vi "json Insert - String Path.vi"(8 "error in (no error)":errorcluster, 9 "anything":variant, 10 "path":string, 11 "JSON Document in":refnum<class "JSON Document.lvclass">) -> (0 "error out":errorcluster, 1 "replaced?":bool, 3 "JSON Document out":refnum<class "JSON Document.lvclass">)   [LabVIEW 2016, in "JSON Document.lvclass"]
uses:
  JSON Document.lvclass
  json query/json Query - string path.vi
  <vilib>/Utility/Data Type/NI_Data Type.lvlib
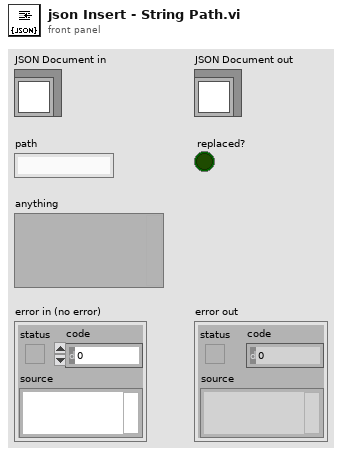
[diagram p1: front panel]
types:
  T1 = typedef "NI_Data Type.lvlib/Data Type.ctl" = enum8{"Invalid Type", "Void", "I8", "I16", "I32", "I64", "U8", "U16", "U32", "U64", "Single Float", "Double Float", "Extended Float", "Single Complex", "Double Complex", "Extended Complex", "Enum U8", "Enum U16", "Enum U32", "Enum U64", "Single Float With Unit", "Double Float With Unit", "Extended Float With Unit", "Single Complex with Unit", "Double Complex with Unit", "Extended Complex with Unit", "Boolean", "String", "Path", "Picture", "Tag", "Array", "Cluster", "Variant", "LV Variant", "Waveform", "Timestamp", "Digital Waveform", "Digital Data", "ExpressData", "Refnum", "External Data", "VI", "Poly VI", "LabVIEW Class Instance", "Fixed Point"}
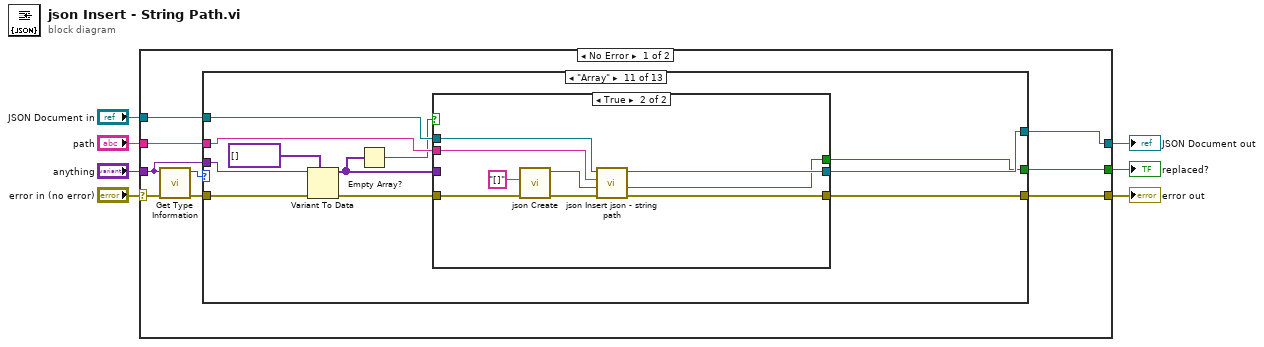
[diagram p0: block diagram]
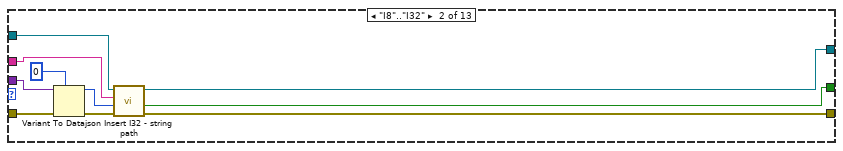
[diagram p3: hidden frame]
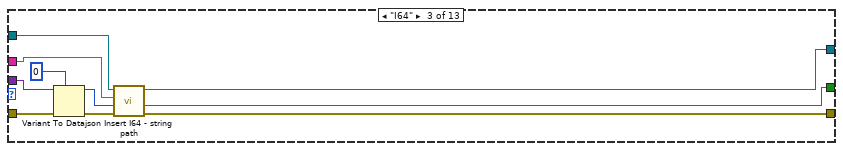
[diagram p4: hidden frame]
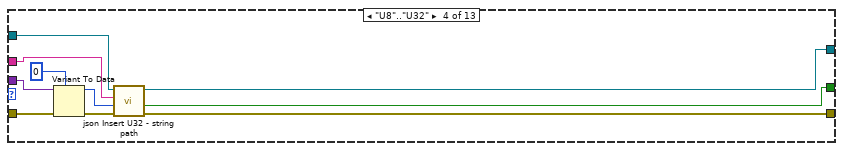
[diagram p5: hidden frame]
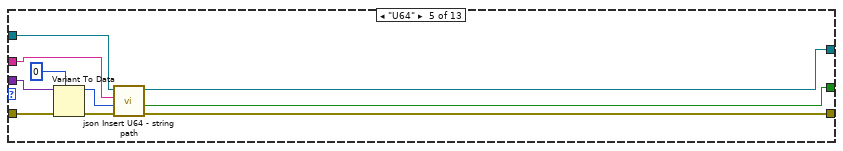
[diagram p6: hidden frame]
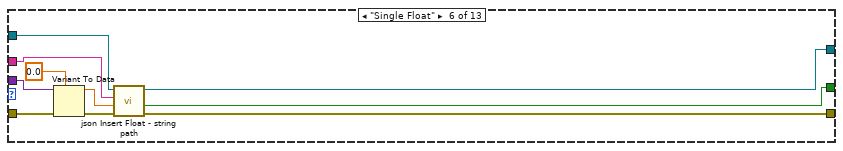
[diagram p7: hidden frame]
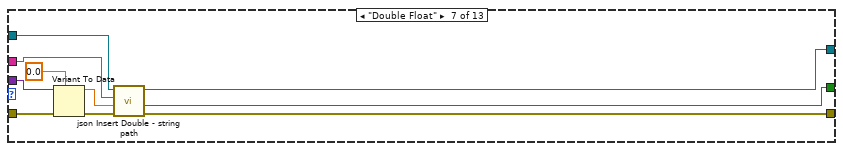
[diagram p8: hidden frame]
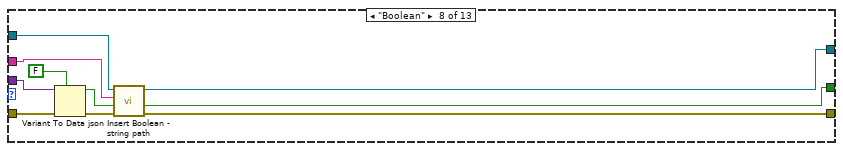
[diagram p9: hidden frame]
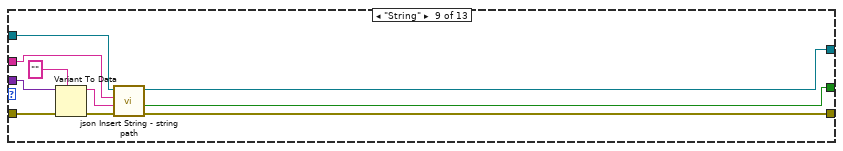
[diagram p10: hidden frame]
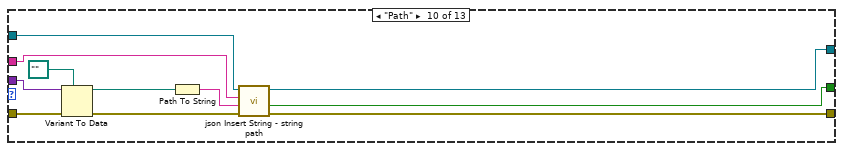
[diagram p11: hidden frame]
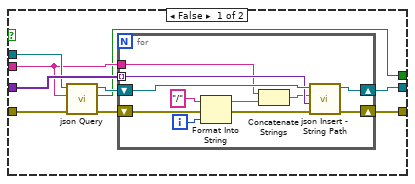
[diagram p12: hidden frame]
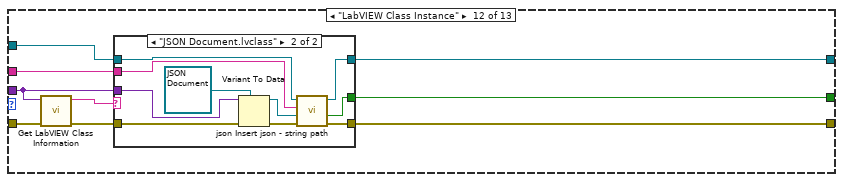
[diagram p13: hidden frame]
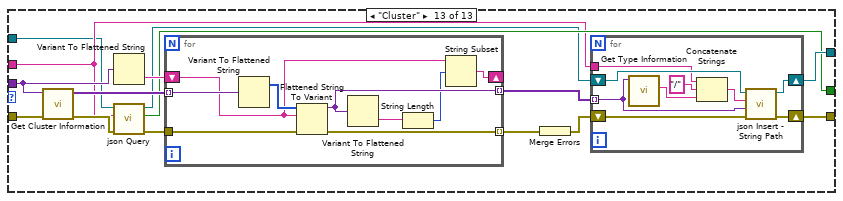
[diagram p15: hidden frame]
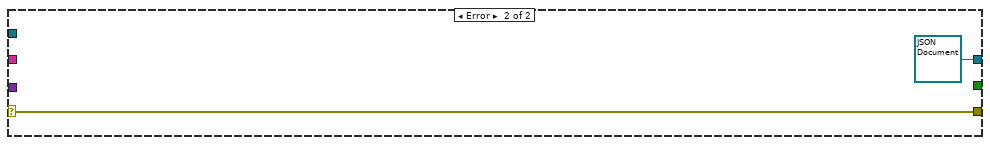
[diagram p16: hidden frame]
diagram:
  n1 = case shown="No Error" "error in (no error)" {
    selector: "error in (no error)" -> [w12 w204]
    tunnel: "anything" -> [w15 _]
    tunnel: [w13 refnum<class "JSON Document.lvclass"> refnum ("JSON Document out")] -> w5
    tunnel: [w11 w204] -> w4
    tunnel: "JSON Document in" -> [w10 _]
    tunnel: "path" -> [w9 _]
    tunnel: [w8 _] -> w1
    frame No Error {
      n2 = call <vilib>:"Get Type Information.vi"("error in (no error)"=w12, "Variant"=w15) -> ("error out"=w14:errorcluster, "Type"=w16:T1)  [unwired: 5 in, 3 out]
      n3 = case shown="\"Array\"" w16 {
        tunnel: w15 -> [_ w27 w37 w47 w57 w67 w77 w87 w97 w108 w119 w156 w182]
        tunnel: w14 -> [w18 w26 w36 w46 w56 w66 w76 w86 w96 w107 w118 w158 w178]
        tunnel: w10 -> [w17 w24 w34 w44 w54 w64 w74 w84 w94 w105 w116 w154 w172]
        tunnel: [w17 w22 w32 w42 w52 w62 w72 w82 w92 w104 w115 w151 w179] -> w13
        tunnel: [w18 w21 w31 w41 w51 w61 w71 w81 w91 w103 w114 w152 w177] -> w11
        tunnel: w9 -> [_ w20 w30 w40 w50 w60 w70 w80 w90 w102 w113 w153 w173]
        tunnel: [_ w19 w29 w39 w49 w59 w69 w79 w89 w101 w110 w150 w174] -> w8
        frame "Invalid Type", Default {
        }
        frame "I8".."I32" {
          n4 = Variant To Data(error in=w26, type=0, Variant=w27) -> (data=w23:i32, error out=w25:errorcluster)
          n5 = call "json Insert I32 - string path.vi"("error in (no error)"=w25, "anything"=w23, "path"=w20, "JSON Document in"=w24) -> ("error out"=w21:errorcluster, "replaced?"=w19:bool, "JSON Document out"=w22:refnum<class "JSON Document.lvclass">)  [unwired: 5 in]
        }
        frame "I64" {
          n6 = Variant To Data(error in=w36, type=i64 0, Variant=w37) -> (data=w33:i64, error out=w35:errorcluster)
          n7 = call "json Insert I64 - string path.vi"("error in (no error)"=w35, "anything"=w33, "path"=w30, "JSON Document in"=w34) -> ("error out"=w31:errorcluster, "replaced?"=w29:bool, "JSON Document out"=w32:refnum<class "JSON Document.lvclass">)  [unwired: 5 in]
        }
        frame "U8".."U32" {
          n8 = Variant To Data(error in=w46, type=u32 0, Variant=w47) -> (data=w43:u32, error out=w45:errorcluster)
          n9 = call "json Insert U32 - string path.vi"("error in (no error)"=w45, "anything"=w43, "path"=w40, "JSON Document in"=w44) -> ("error out"=w41:errorcluster, "replaced?"=w39:bool, "JSON Document out"=w42:refnum<class "JSON Document.lvclass">)  [unwired: 5 in]
        }
        frame "U64" {
          n10 = Variant To Data(error in=w56, type=u64 0, Variant=w57) -> (data=w53:u64, error out=w55:errorcluster)
          n11 = call "json Insert U64 - string path.vi"("error in (no error)"=w55, "anything"=w53, "path"=w50, "JSON Document in"=w54) -> ("error out"=w51:errorcluster, "replaced?"=w49:bool, "JSON Document out"=w52:refnum<class "JSON Document.lvclass">)  [unwired: 5 in]
        }
        frame "Single Float" {
          n12 = Variant To Data(error in=w66, type=sgl 0.0, Variant=w67) -> (data=w63:sgl, error out=w65:errorcluster)
          n13 = call "json Insert Float - string path.vi"("error in (no error)"=w65, "anything"=w63, "path"=w60, "JSON Document in"=w64) -> ("error out"=w61:errorcluster, "replaced?"=w59:bool, "JSON Document out"=w62:refnum<class "JSON Document.lvclass">)  [unwired: 5 in]
        }
        frame "Double Float" {
          n14 = Variant To Data(error in=w76, type=0.0, Variant=w77) -> (data=w73:dbl, error out=w75:errorcluster)
          n15 = call "json Insert Double - string path.vi"("error in (no error)"=w75, "anything"=w73, "path"=w70, "JSON Document in"=w74) -> ("error out"=w71:errorcluster, "replaced?"=w69:bool, "JSON Document out"=w72:refnum<class "JSON Document.lvclass">)  [unwired: 5 in]
        }
        frame "Boolean" {
          n16 = Variant To Data(error in=w86, type=FALSE, Variant=w87) -> (data=w83:bool, error out=w85:errorcluster)
          n17 = call "json Insert Boolean - string path.vi"("error in (no error)"=w85, "anything"=w83, "path"=w80, "JSON Document in"=w84) -> ("error out"=w81:errorcluster, "replaced?"=w79:bool, "JSON Document out"=w82:refnum<class "JSON Document.lvclass">)  [unwired: 5 in]
        }
        frame "String" {
          n18 = Variant To Data(error in=w96, type="", Variant=w97) -> (data=w93:string, error out=w95:errorcluster)
          n19 = call "json Insert String - string path.vi"("error in (no error)"=w95, "anything"=w93, "path"=w90, "JSON Document in"=w94) -> ("error out"=w91:errorcluster, "replaced?"=w89:bool, "JSON Document out"=w92:refnum<class "JSON Document.lvclass">)  [unwired: 5 in]
        }
        frame "Path" {
          n20 = Variant To Data(error in=w107, type=path "", Variant=w108) -> (data=w99:path, error out=w106:errorcluster)
          n21 = Path To String(path=w99) -> (string=w100:string)
          n22 = call "json Insert String - string path.vi"("error in (no error)"=w106, "anything"=w100, "path"=w102, "JSON Document in"=w105) -> ("error out"=w103:errorcluster, "replaced?"=w101:bool, "JSON Document out"=w104:refnum<class "JSON Document.lvclass">)  [unwired: 5 in]
        }
        frame "Array" {
          n23 = Variant To Data(error in=w118, type=variant[] [], Variant=w119) -> (data=w111:variant[], error out=w117:errorcluster)
          n24 = Empty Array?(array=w111) -> (empty?=w112:bool)
          n25 = case shown="True" w112 {
            tunnel: w117 -> [w122 w149]
            tunnel: w116 -> [w126 w148]
            tunnel: w111 -> [w129 _]
            tunnel: [w128 w147] -> w115
            tunnel: [w127 w146] -> w114
            tunnel: w113 -> [w124 w145]
            tunnel: [w123 w141] -> w110
            frame False {
              n26 = call-poly "json Query.vi"("error in (no error)"=w122, "path"=w124, "JSON Document in"=w126) -> ("error out"=w121:errorcluster, "found?"=w123:bool, "JSON Document out"=w125:refnum<class "JSON Document.lvclass">)  [unwired: 5 in, 1 out]
              n27 = for {
                tunnel: w129 -> [w137] mode=indexing
                shift-right: [w139] -> w127
                shift-left: w121 -> [w131]
                shift-right: [w140] -> w128
                shift-left: w125 -> [w138]
                tunnel: w124 -> [w134]
                i -> [w136]
                n28 = Format Into String(initial string="/", error in=w131, w136) -> (resulting string=w133:string, error out=w130:errorcluster)  [unwired: 1 in]
                n29 = Concatenate Strings(w134, w133) -> (w132:string)
                n30 = call "json Insert - String Path.vi"("error in (no error)"=w130, "anything"=w137, "path"=w132, "JSON Document in"=w138) -> ("error out"=w139:errorcluster, "JSON Document out"=w140:refnum<class "JSON Document.lvclass">)  [unwired: 5 in, 1 out]
              }
            }
            frame True {
              n31 = call "json Create.vi"("error in (no error)"=w149, "JSON String"="[]") -> ("error out"=w143:errorcluster, "JSON Document out"=w144:refnum<class "JSON Document.lvclass">)  [unwired: 8 in]
              n32 = call "json Insert json - string path.vi"("error in (no error)"=w143, "anything"=w144, "path"=w145, "JSON Document in"=w148) -> ("error out"=w146:errorcluster, "replaced?"=w141:bool, "JSON Document out"=w147:refnum<class "JSON Document.lvclass">)  [unwired: 5 in]
            }
          }
        }
        frame "LabVIEW Class Instance" {
          n33 = call <vilib>:"Get LabVIEW Class Information.vi"("error in (no error)"=w158, "Variant"=w156) -> ("error out"=w155:errorcluster, "LabVIEW Class File Name"=w157:string)  [unwired: 7 in, 1 out]
          n34 = case shown="\"JSON Document.lvclass\"" w157 {
            tunnel: w156 -> [_ w170]
            tunnel: w155 -> [w159 w168]
            tunnel: w154 -> [w160 w167]
            tunnel: w153 -> [_ w166]
            tunnel: [w159 w163] -> w152
            tunnel: [w160 w162] -> w151
            tunnel: [_ w161] -> w150
            frame "False", Default {
            }
            frame "JSON Document.lvclass" {
              n35 = Variant To Data(error in=w168, type=refnum<class "JSON Document.lvclass"> refnum ("JSON Document in"), Variant=w170) -> (data=w165:refnum<class "JSON Document.lvclass">, error out=w164:errorcluster)
              n36 = call "json Insert json - string path.vi"("error in (no error)"=w164, "anything"=w165, "path"=w166, "JSON Document in"=w167) -> ("error out"=w163:errorcluster, "replaced?"=w161:bool, "JSON Document out"=w162:refnum<class "JSON Document.lvclass">)  [unwired: 5 in]
            }
          }
        }
        frame "Cluster" {
          n37 = call <vilib>:"Get Cluster Information.vi"("error in (no error)"=w178, "Variant"=w182) -> ("error out"=w176:errorcluster, "Cluster Elements"=w184:variant[])  [unwired: 8 in]
          n38 = Variant To Flattened String(Variant=w182) -> (data string=w185:string)  [unwired: 1 out]
          n39 = call-poly "json Query.vi"("error in (no error)"=w176, "path"=w173, "JSON Document in"=w172) -> ("error out"=w175:errorcluster, "found?"=w174:bool, "JSON Document out"=w171:refnum<class "JSON Document.lvclass">)  [unwired: 5 in, 1 out]
          n40 = for {
            tunnel: w184 -> [w203] mode=indexing
            tunnel: [w201] -> w181 mode=indexing
            shift-right: [w197] -> _
            shift-left: w185 -> [w200]
            tunnel: w175 -> [w196]
            tunnel: [w195] -> w183 mode=indexing
            n41 = Variant To Flattened String(Variant=w203) -> (1:w202:i16[])  [unwired: 1 out]
            n42 = Flattened String To Variant(4:w196, 6:w200, 7:w202) -> (0:w195:errorcluster, 3:w201:variant)
            n43 = Variant To Flattened String(Variant=w201) -> (data string=w199:string)  [unwired: 1 out]
            n44 = String Length(string=w199) -> (length=w198:i32)
            n45 = String Subset(string=w200, offset (0)=w198) -> (substring=w197:string)  [unwired: 1 in]
          }
          n46 = Merge Errors(w183) -> (w180:errorcluster)
          n47 = for {
            tunnel: w181 -> [w188] mode=indexing
            shift-right: [w193] -> w179
            shift-left: w171 -> [w194]
            tunnel: w173 -> [w192]
            shift-right: [w186] -> w177
            shift-left: w180 -> [w187]
            n48 = call <vilib>:"Get Type Information.vi"("Variant"=w188) -> ("Name"=w190:string)  [unwired: 6 in, 4 out]
            n49 = Concatenate Strings(w192, "/" ("string"), w190) -> (w189:string)
            n50 = call "json Insert - String Path.vi"("error in (no error)"=w187, "anything"=w188, "path"=w189, "JSON Document in"=w194) -> ("error out"=w186:errorcluster, "JSON Document out"=w193:refnum<class "JSON Document.lvclass">)  [unwired: 5 in, 1 out]
          }
        }
      }
    }
    frame Error {
    }
  }
  "error out" <- w4
  "JSON Document out" <- w5
  "replaced?" <- w1
